vi "ServoFollowLight.vi"() -> ()   [LabVIEW 2019]
uses:
  <vilib>/LabVIEW Interface for Arduino/Type Defs/Board Type.ctl
  <vilib>/LabVIEW Interface for Arduino/LabVIEW Interface for Arduino.lvlib
panel:
  in  "coef":dbl=1.0
  in  "balance":dbl(slide) scale=-3.0..10.0
  in  "2":u8=1
  in  "1":u8
  out "Waveform Chart":T1(graph)={"Light Intensity (0 - 100)"=47.922000000000004, "Light Intensity (0 - 100)"=40.278000000000006, -7.643999999999998}
  out "U2":dbl=40.278000000000006
  out "U1":dbl=47.922000000000004
  in  "milliseconds to wait":u32=50
  out "error out":errorcluster={"status"=FALSE, "code"=1073676294, "source"="VISA Read in LabVIEW Interface for Arduino.lvlib:Send Receive.vi->LabVIEW Interface for Arduino.lvlib:Analog Read Pin.vi->LabVIEW Interface for Arduino.lvlib:Photocell Read.vi->Untitled 23"}
  in  "VISA resource":refnum<visa-resource-name>="COM4"
  in  "stop":bool
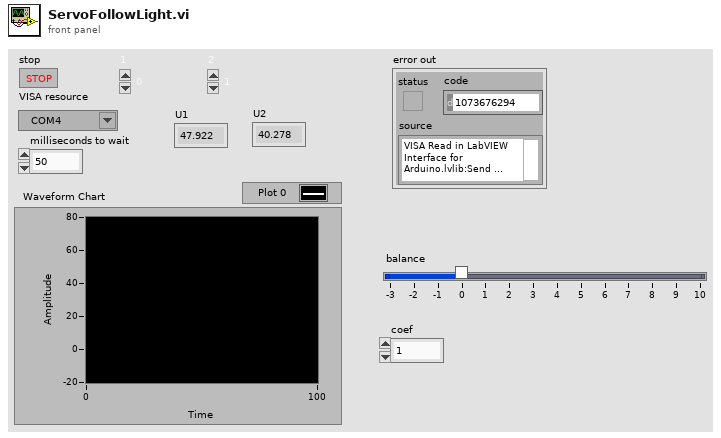
[diagram p1: front panel]
types:
  T1 = cluster{"Light Intensity (0 - 100)":dbl, "Light Intensity (0 - 100)":dbl, dbl}
  T2 = typedef "LabVIEW Interface for Arduino.lvlib/Board Type.ctl" = enum16{"Uno", "Dimuelanove w/Atmega 328", "Mega 2560"}
  T3 = typedef "LabVIEW Interface for Arduino.lvlib/Arduino Resource.ctl" = cluster{"VISA resource":refnum<visa-resource-name>, "Board Type":T2, "Connection Type":enum8{"USB / Serial"}, "Bytes Per Packet (15)":u8}
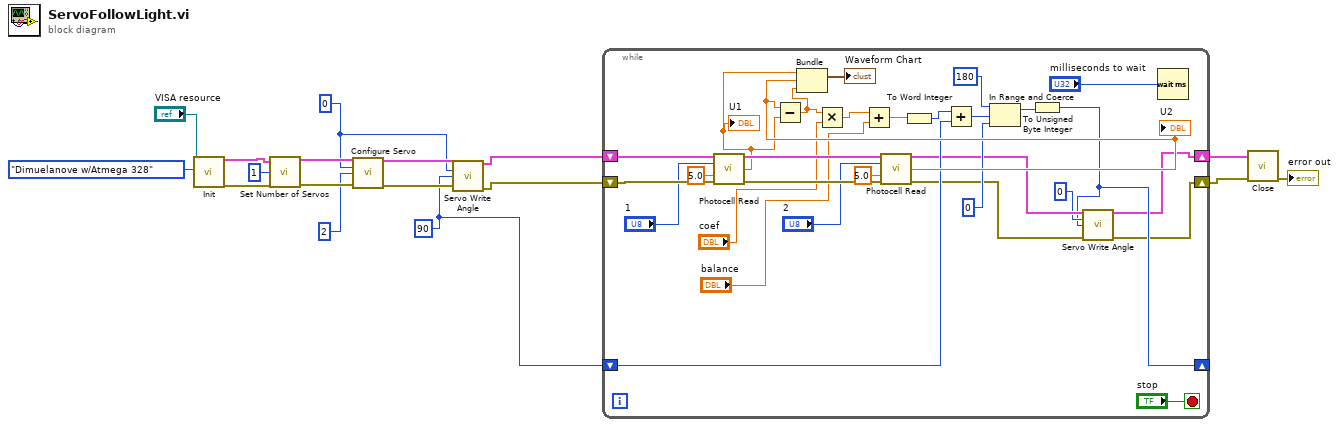
[diagram p0: block diagram]
diagram:
  w1 = u8 90 ("Angle (Degrees)")
  w4 = u8 0 ("Servo Number (0)")
  n1 = call <vilib>:"Init.vi"("VISA resource"="VISA resource", "Board Type (Uno)"=Board_Type."Dimuelanove w/Atmega 328") -> ("Arduino Resource"=w11:T3, "error out"=w10:errorcluster)  [unwired: 16 in]
  n2 = call <vilib>:"Set Number of Servos.vi"("Arduino Resource"=w11, "Number Of Servos (1)"=u8 1, "error in"=w10) -> ("Arduino Resource"=w9:T3, "error out"=w8:errorcluster)  [unwired: 11 in]
  n3 = call <vilib>:"Configure Servo.vi"("Arduino Resource"=w9, "Servo Number (0)"=w4, "DIO Pin (2)"=u8 2, "error in"=w8) -> ("Arduino Resource"=w6:T3, "error out"=w5:errorcluster)  [unwired: 10 in]
  n4 = call <vilib>:"Servo Write Angle.vi"("Arduino Resource"=w6, "Servo Number"=w4, "Angle (Degrees)"=w1, "error in"=w5) -> ("Arduino Resource"=w3:T3, "error out"=w2:errorcluster)  [unwired: 10 in]
  n5 = while {
    shift-right: [w18] -> w14
    shift-left: w2 -> [w44]
    shift-right: [w19] -> w15
    shift-left: w3 -> [w45]
    shift-right: [w20] -> _
    shift-left: w1 -> [w29]
    stop <- "stop" stop-if-true
    n6 = call <vilib>:"Photocell Read.vi"("Arduino Resource"=w45, "Photo Cell Pin (0)"="1", "Vcc (5)"=5.0, "error in"=w44) -> ("Arduino Resource"=w43:T3, "Light Intensity (0 - 100)"=w35:dbl, "error out"=w42:errorcluster)  [unwired: 9 in]
    "U1" <- w35
    n7 = call <vilib>:"Photocell Read.vi"("Arduino Resource"=w43, "Photo Cell Pin (0)"="2", "Vcc (5)"=5.0, "error in"=w42) -> ("Arduino Resource"=w23:T3, "Light Intensity (0 - 100)"=w36:dbl, "error out"=w22:errorcluster)  [unwired: 9 in]
    "U2" <- w36
    n8 = Subtract(x=w36, y=w35) -> (x-y=w34:dbl)
    n9 = Bundle("Light Intensity (0 - 100)"=w35, "Light Intensity (0 - 100)"=w36, w34) -> (→"Waveform Chart":T1)  [unwired: 1 in]
    n10 = Multiply(x=w34, y="coef") -> (x*y=w32:dbl)
    n11 = Add(x=w32, y="balance") -> (x+y=w30:dbl)
    n12 = To Word Integer(number=w30) -> (16bit integer=w28:i16)
    n13 = Add(x=w28, y=w29) -> (x+y=w27:i16)
    n14 = In Range and Coerce(upper limit=i16 180, x=w27, lower limit=i16 0) -> (coerced(x)=w24:i16)  [unwired: 1 out]
    n15 = To Unsigned Byte Integer(number=w24) -> (unsigned 8bit integer=w20:u8)
    n16 = call <vilib>:"Servo Write Angle.vi"("Arduino Resource"=w23, "Servo Number"=u8 0, "Angle (Degrees)"=w20, "error in"=w22) -> ("Arduino Resource"=w19:T3, "error out"=w18:errorcluster)  [unwired: 10 in]
    n17 = Wait (ms)(milliseconds to wait="milliseconds to wait") -> ()  [unwired: 1 out]
  }
  n18 = call <vilib>:"Close.vi"("Arduino Resource"=w15, "error in"=w14) -> ("error out"=→"error out":errorcluster)  [unwired: 13 in]
